vi "Exercise 4.6.vi"() -> ()   [LabVIEW 2020]
panel:
  in  "Left":i32(slide)=90 min=0 max=180 scale=0.0..180.0
  out "Read Position\nLeft":string
  in  "Right":i32(slide)=90 scale=-20.0..200.0
  out "Read Position\nRight":string
  in  "Center":i32(slide)=90 min=0 max=180 scale=0.0..180.0
  out "Read Position\nCenter":string
  out "Read Position\n Jaw":string
  in  "stop":bool
  in  "Jaw":i32(slide)=90 min=90 scale=90.0..180.0
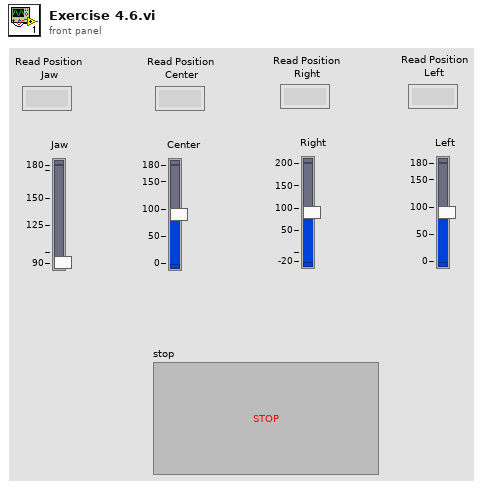
[diagram p1: front panel]
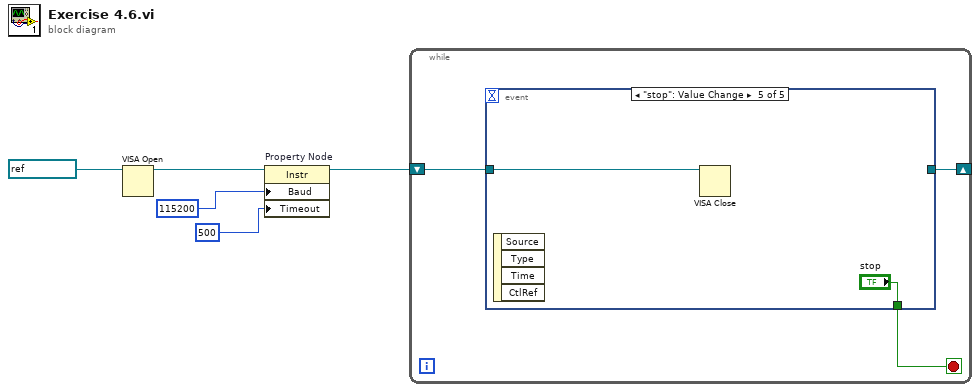
[diagram p0: block diagram]
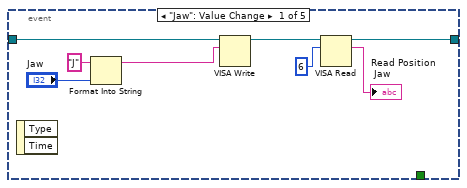
[diagram p2: hidden frame]
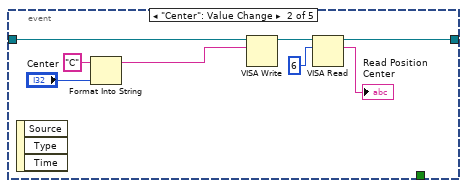
[diagram p3: hidden frame]
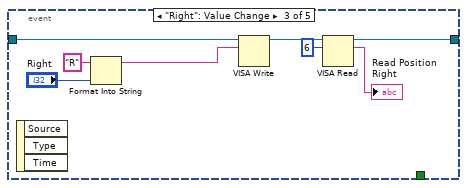
[diagram p4: hidden frame]
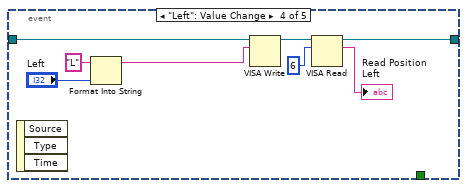
[diagram p5: hidden frame]
diagram:
  n1 = VISA Open(VISA resource name=refnum<visa-resource-name> "COM13") -> (VISA resource name=w4:refnum<visa-resource-name>)  [unwired: 4 in, 1 out]
  n2 = property on="Property Node" class="Instr"(reference=w4, "Baud"=u32 115200 ("Serial Settings:Baud Rate"), "Timeout"=u32 500 ("General Settings:Timeout Value")) -> (reference out=w2:refnum<visa-resource-name>)  [unwired: 1 in, 1 out]
  n3 = while {
    shift-right: [w7] -> _
    shift-left: w2 -> [w8]
    stop <- w6 stop-if-true
    n4 = event shown="[4] \"stop\": Value Change" {
      selector: _ -> [_ _ _ _ _]
      dyn-events: _ -> [_ _ _ _ _]
      timeout: _ -> [_ _ _ _ _]
      tunnel: w8 -> [w16 w24 w32 w40 w42]
      tunnel: [w11 w19 w28 w35 _] -> w7
      tunnel: [_ _ _ _ "stop"] -> w6
      event "Jaw": Value Change {
        n5 = event-data() -> ()  [unwired: 1 in, 2 out]
        n6 = Format Into String "Format Into String"(initial string="J", "Jaw") -> (resulting string=w13:string)  [unwired: 2 in, 1 out]
        n7 = VISA Write(VISA resource name=w16, write buffer=w13) -> (VISA resource name out=w12:refnum<visa-resource-name>)  [unwired: 1 in, 2 out]
        n8 = VISA Read(VISA resource name=w12, byte count=u32 6) -> (VISA resource name out=w11:refnum<visa-resource-name>, read buffer=→"Read Position\n Jaw":string)  [unwired: 1 in, 2 out]
      }
      event "Center": Value Change {
        n9 = event-data() -> ()  [unwired: 1 in, 3 out]
        n10 = Format Into String "Format Into String"(initial string="C", "Center") -> (resulting string=w21:string)  [unwired: 2 in, 1 out]
        n11 = VISA Write(VISA resource name=w24, write buffer=w21) -> (VISA resource name out=w20:refnum<visa-resource-name>)  [unwired: 1 in, 2 out]
        n12 = VISA Read(VISA resource name=w20, byte count=u32 6) -> (VISA resource name out=w19:refnum<visa-resource-name>, read buffer=→"Read Position\nCenter":string)  [unwired: 1 in, 2 out]
      }
      event "Right": Value Change {
        n13 = event-data() -> ()  [unwired: 1 in, 3 out]
        n14 = Format Into String "Format Into String"(initial string="R", "Right") -> (resulting string=w29:string)  [unwired: 2 in, 1 out]
        n15 = VISA Write(VISA resource name=w32, write buffer=w29) -> (VISA resource name out=w26:refnum<visa-resource-name>)  [unwired: 1 in, 2 out]
        n16 = VISA Read(VISA resource name=w26, byte count=u32 6) -> (VISA resource name out=w28:refnum<visa-resource-name>, read buffer=→"Read Position\nRight":string)  [unwired: 1 in, 2 out]
      }
      event "Left": Value Change {
        n17 = event-data() -> ()  [unwired: 1 in, 3 out]
        n18 = Format Into String "Format Into String"(initial string="L", "Left") -> (resulting string=w37:string)  [unwired: 2 in, 1 out]
        n19 = VISA Write(VISA resource name=w40, write buffer=w37) -> (VISA resource name out=w36:refnum<visa-resource-name>)  [unwired: 1 in, 2 out]
        n20 = VISA Read(VISA resource name=w36, byte count=u32 6) -> (VISA resource name out=w35:refnum<visa-resource-name>, read buffer=→"Read Position\nLeft":string)  [unwired: 1 in, 2 out]
      }
      event "stop": Value Change {
        n21 = event-data() -> ()  [unwired: 1 in, 4 out]
        n22 = VISA Close(VISA resource name=w42) -> ()  [unwired: 1 in, 1 out]
      }
    }
  }
